vi "Line Datum.vi"(0 "Image in":T2, 1 "Small FOV?":bool, 2 "Angle of rotation":dbl, 3 "half Datum arrow width( in pixels)":u16=50, 4 "Arrow height (in pixels)":u16=50, 5 "Datum origin":cluster{"X":sgl, "Y":sgl}, 6 "Start index":i32=6, 7 "error in (no error)":errorcluster, 8 "Color":u32, 9 "Datum line angle":dbl, 10 "Box start index":i32=1, 12 "sleeping line length(in pixels)":u16=75, 13 "Angular line length(in pixels)":u16=150, 14 "pixel factor":dbl=29160000.0, 15 "Reference string":string="ZAMP", 16 "Measurement name":string, 17 "Fixed overlay details":T1={"Overlay coordinates"=[], "Config coordinates"=[], "Inspection mode?"=TRUE}) -> (20 "Image out":T2, 21 "Text origin out":cluster{"X":sgl, "Y":sgl}, 23 "Overlay coordinates out":cluster{"X":dbl, "Y":dbl}[](array[cluster]), 27 "error out":errorcluster)   [LabVIEW 2019]
uses:
  <vilib>/vision/Image Controls.llb/IMAQ Image.ctl
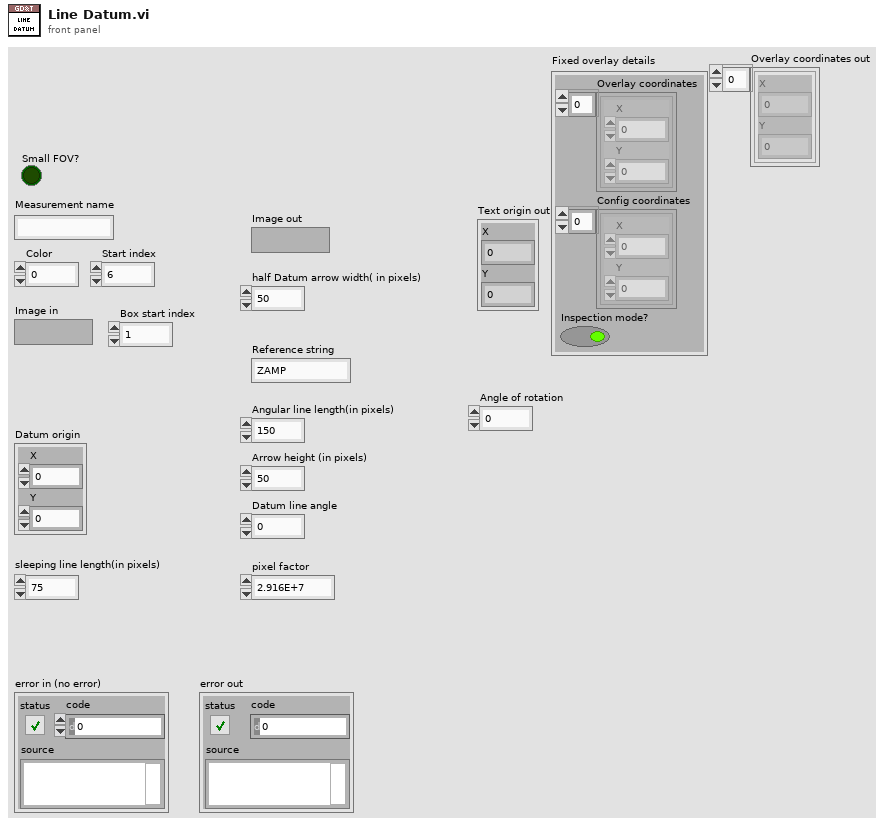
[diagram p1: front panel]
types:
  T1 = cluster{"Overlay coordinates":cluster{"X":dbl, "Y":dbl}[], "Config coordinates":cluster{"X":dbl, "Y":dbl}[], "Inspection mode?":bool}
  T2 = typedef "IMAQ Image.ctl" = refnum<image>
  T3 = enum16{"User-specified Font", "Application Font", "System Font", "Dialog Font"}
  T4 = cluster{"Desired Font (Application)":enum16{"User-specified Font", "Application Font", "System Font", "Dialog Font"}, "[User-specified Font]":cluster{"Font Name":string, "Size":i16, "Strikeout?":bool, "Italic?":bool, "Underline?":bool, "Outline?":bool, "Shadow?":bool, "Bold?":bool, "Rotation Angle":dbl}, "Horizontal Alignment":i16, "Vertical Alignment":i16}
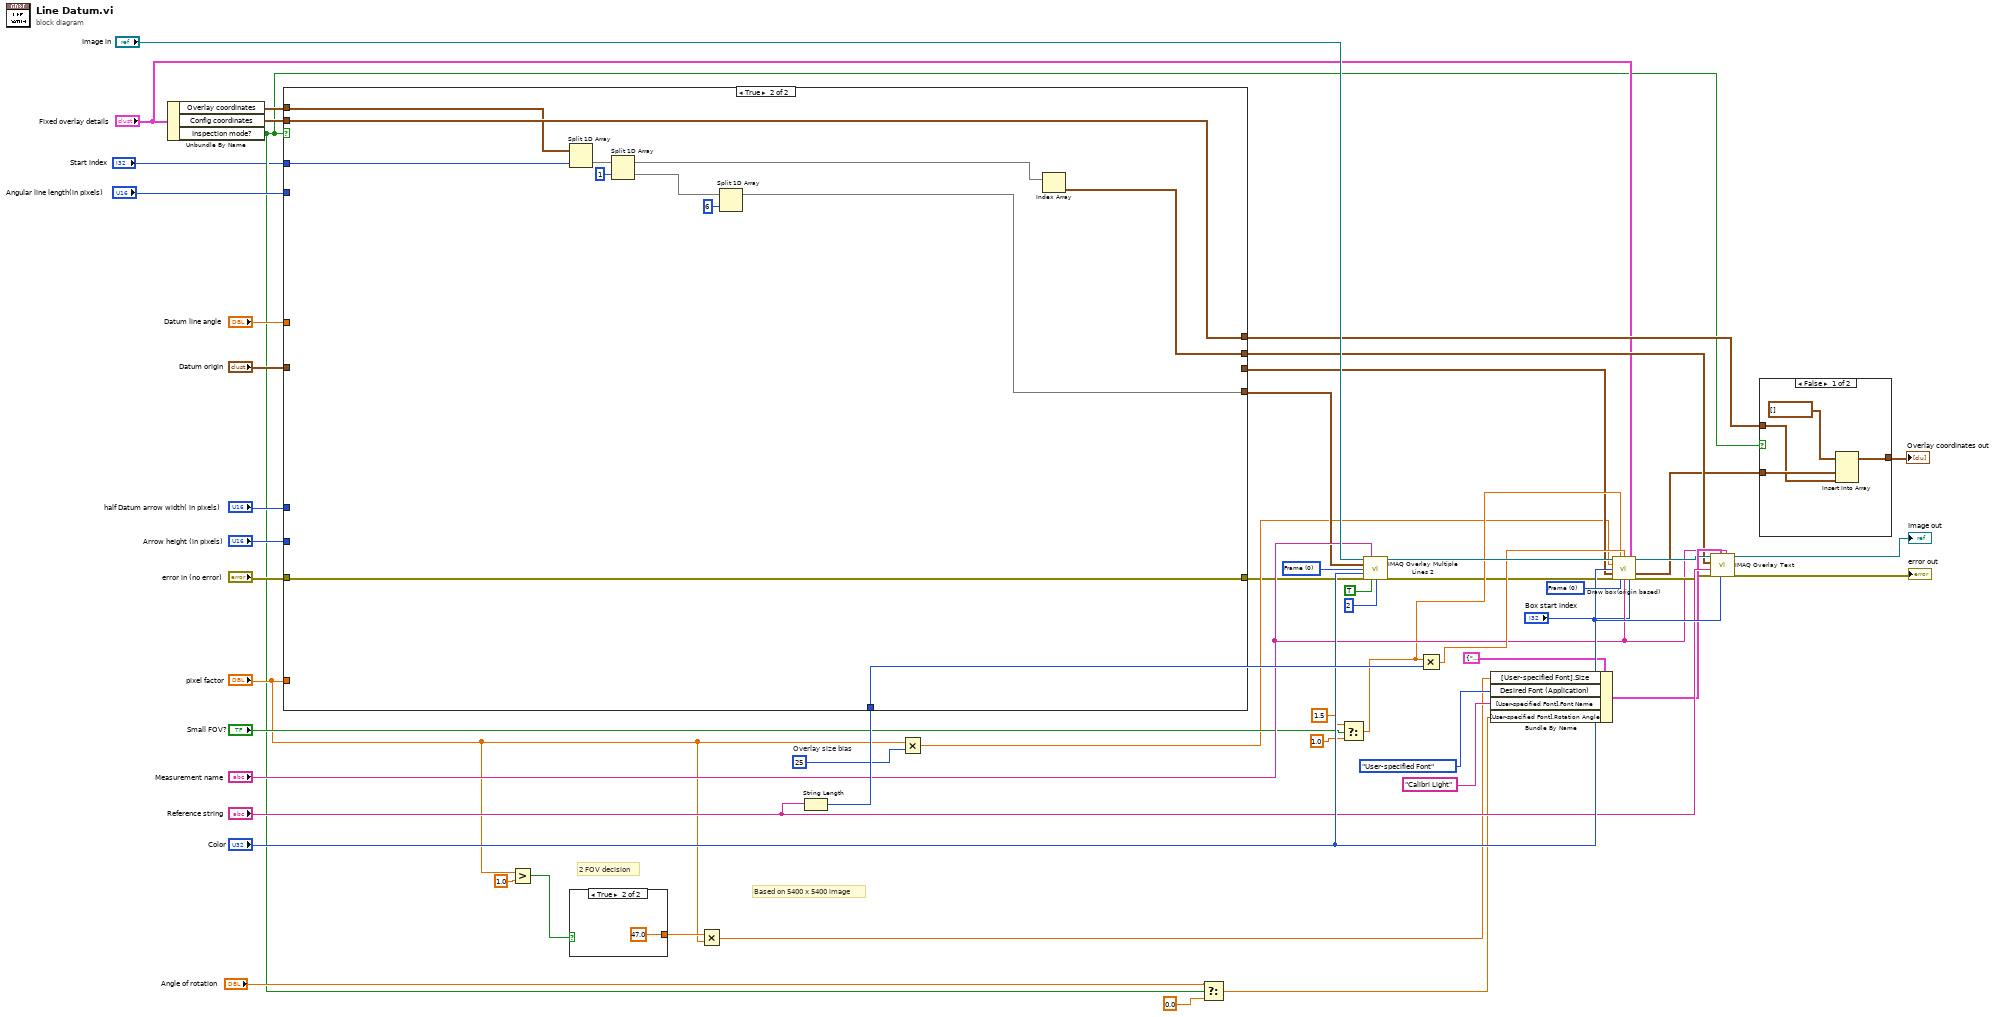
[diagram p0: block diagram]
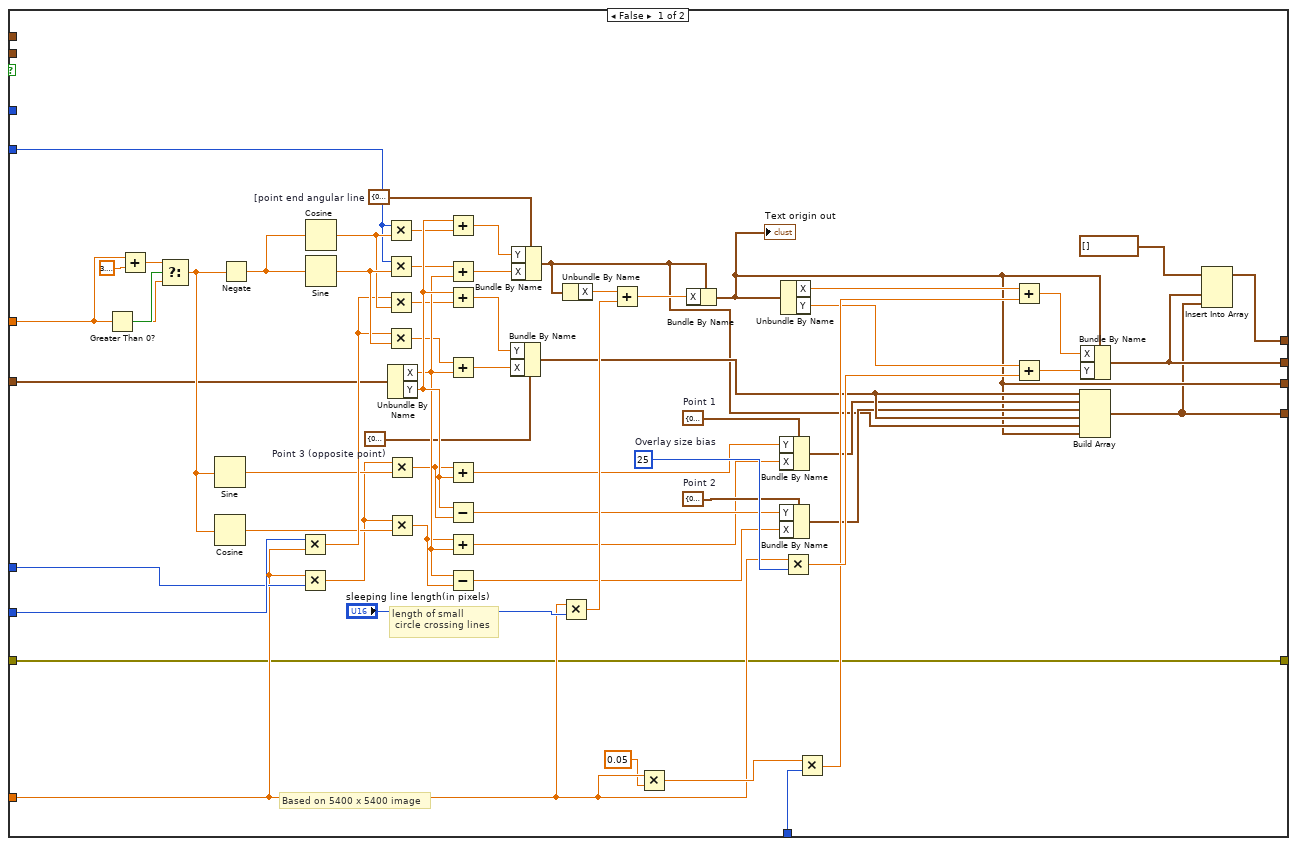
[diagram p3: hidden frame]
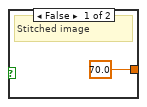
[diagram p4: hidden frame]
diagram:
  w14 = u16 25  # Overlay size bias
  w50 = u32 0 items=["Frame", "Fill"] ("Drawing Mode (Frame)")
  w38 = u32 0 items=["Frame", "Fill"] ("Drawing Mode (Frame)")
  # "2 FOV decision"
  # "Based on 5400 x 5400 image"
  n1 = Unbundle By Name("Fixed overlay details") -> ("Overlay coordinates"=w17:cluster{"X":dbl, "Y":dbl}[], "Config coordinates"=w16:cluster{"X":dbl, "Y":dbl}[], "Inspection mode?"=w4:bool)
  n2 = Greater?(x="pixel factor", y=1.0) -> (0:w35:bool)
  n3 = case shown="True" w35 {
    tunnel: [70.0 ("x") 47.0 ("x")] -> w34
    frame False {
      # "Stitched image"
    }
    frame True {
    }
  }
  n4 = Multiply(x=w34, y="pixel factor") -> (x*y=w28:dbl)
  n5 = String Length(string="Reference string") -> (length=w53:i32)
  n6 = case shown="True" w4 {
    tunnel: w53 -> [w108 _]
    tunnel: "Arrow height (in pixels)" -> [w82 _]
    tunnel: "half Datum arrow width( in pixels)" -> [w80 _]
    tunnel: "Datum origin" -> [w70 _]
    tunnel: "pixel factor" -> [w69 _]
    tunnel: "Angular line length(in pixels)" -> [w68 _]
    tunnel: "Datum line angle" -> [w67 _]
    tunnel: [w56 w119] -> w21
    tunnel: [w59 _] -> w20
    tunnel: [w61 w118] -> w19
    tunnel: w17 -> [_ w126]
    tunnel: w16 -> [_ w127]
    tunnel: [w58 w127] -> w11
    tunnel: "error in (no error)" -> [w57 w123]
    tunnel: [w57 w123] -> w8
    tunnel: "Start index" -> [_ w117]
    frame False {
      w116 = u16 25  # Overlay size bias
      w90 = cluster{"X":sgl, "Y":sgl} {"X"=0.0, "Y"=0.0}  # [point end angular line
      w79 = cluster{"X":sgl, "Y":sgl} {"X"=0.0, "Y"=0.0}  # Point 3 (opposite point)
      w76 = cluster{"X":sgl, "Y":sgl} {"X"=0.0, "Y"=0.0}  # Point 2
      w71 = cluster{"X":sgl, "Y":sgl} {"X"=0.0, "Y"=0.0}  # Point 1
      # "Based on 5400 x 5400 image"
      # "length of small\n circle crossing lines"
      n7 = Greater Than 0?(x=w67) -> (x > 0?=w114:bool)
      n8 = Add(x=w67, y=3.141592653589793) -> (x+y=w112:dbl)
      n9 = Select(t=w112, s=w114, f=w67) -> (s? t:f=w113:dbl)
      n10 = Sine(x=w113) -> (sin(x)=w88:dbl)
      n11 = Cosine(x=w113) -> (cos(x)=w87:dbl)
      n12 = Negate(x=w113) -> (-x=w89:dbl)
      n13 = Multiply(x=w82, y=w69) -> (x*y=w93:dbl)
      n14 = Multiply(x=w69, y=w80) -> (x*y=w81:dbl)
      n15 = Cosine(x=w89) -> (cos(x)=w100:dbl)
      n16 = Sine(x=w89) -> (sin(x)=w101:dbl)
      n17 = Multiply(x=w68, y=w100) -> (x*y=w91:dbl)
      n18 = Multiply(x=w68, y=w101) -> (x*y=w92:dbl)
      n19 = Multiply(x=w93, y=w100) -> (x*y=w86:dbl)
      n20 = Multiply(x=w93, y=w101) -> (x*y=w84:dbl)
      n21 = Multiply(x=w81, y=w88) -> (x*y=w74:dbl)
      n22 = Multiply(x=w81, y=w87) -> (x*y=w75:dbl)
      n23 = Unbundle By Name(w70) -> ("X"=w94:sgl, "Y"=w95:sgl)
      n24 = Add(x=w95, y=w91) -> (x+y=w96:dbl)
      n25 = Add(x=w92, y=w94) -> (x+y=w97:dbl)
      n26 = Add(x=w95, y=w86) -> (x+y=w83:dbl)
      n27 = Add(x=w84, y=w94) -> (x+y=w85:dbl)
      n28 = Add(x=w74, y=w95) -> (x+y=w72:dbl)
      n29 = Subtract(x=w95, y=w74) -> (x-y=w78:dbl)
      n30 = Add(x=w75, y=w94) -> (x+y=w73:dbl)
      n31 = Subtract(x=w94, y=w75) -> (x-y=w77:dbl)
      n32 = Bundle By Name(cluster=w79, "Y"=w83, "X"=w85) -> (w65:cluster{"X":sgl, "Y":sgl})
      n33 = Bundle By Name(cluster=w90, "Y"=w96, "X"=w97) -> (w62:cluster{"X":sgl, "Y":sgl})
      n34 = Multiply(x=w69, y="sleeping line length(in pixels)") -> (x*y=w103:dbl)
      n35 = Unbundle By Name(w62) -> ("X"=w99:sgl)
      n36 = Add(x=w99, y=w103) -> (x+y=w102:dbl)
      n37 = Multiply(x=w69, y=0.05) -> (x*y=w109:dbl)
      n38 = Bundle By Name(cluster=w62, "X"=w102) -> (w59:cluster{"X":sgl, "Y":sgl})
      "Text origin out" <- w59
      n39 = Bundle By Name(cluster=w71, "Y"=w72, "X"=w73) -> (w64:cluster{"X":sgl, "Y":sgl})
      n40 = Bundle By Name(cluster=w76, "Y"=w78, "X"=w77) -> (w63:cluster{"X":sgl, "Y":sgl})
      n41 = Unbundle By Name(w59) -> ("X"=w104:sgl, "Y"=w106:sgl)
      n42 = Multiply(x=w69, y=w116) -> (x*y=w115:dbl)
      n43 = Multiply(x=w109, y=w108) -> (x*y=w110:dbl)
      n44 = Add(x=w104, y=w110) -> (x+y=w105:dbl)
      n45 = Add(x=w106, y=w115) -> (x+y=w107:dbl)
      n46 = Build Array(w65, w64, w63, w65, w62, w59) -> (w56:cluster{"X":sgl, "Y":sgl}[])
      n47 = Bundle By Name(cluster=w59, "X"=w105, "Y"=w107) -> (w61:cluster{"X":sgl, "Y":sgl})
      n48 = Insert Into Array(array=cluster{"X":sgl, "Y":sgl}[] [], new element #1=w61, new element #2=w56) -> (w58:cluster{"X":sgl, "Y":sgl}[])  [unwired: 1 in]
    }
    frame True {
      n49 = Split 1D Array(array=w126, index=w117) -> (second subarray=w125:cluster{"X":dbl, "Y":dbl}[])  [unwired: 1 out]
      n50 = Split 1D Array(array=w125, index=1) -> (first subarray=w124:cluster{"X":dbl, "Y":dbl}[], second subarray=w121:cluster{"X":dbl, "Y":dbl}[])
      n51 = Split 1D Array(array=w121, index=6) -> (first subarray=w119:cluster{"X":dbl, "Y":dbl}[])  [unwired: 1 out]
      n52 = Index Array(array=w124) -> (element=w118:cluster{"X":dbl, "Y":dbl})  [unwired: 1 in]
    }
  }
  n53 = Multiply(x="pixel factor", y=w14) -> (x*y=w13:dbl)
  n54 = Select(t="Angle of rotation", s=w4, f=0.0) -> (s? t:f=w5:dbl)
  n55 = Select(t=1.5, s="Small FOV?", f=1.0 ("Width factor")) -> (s? t:f=w22:dbl)
  n56 = call "IMAQ Overlay Multiple Lines 2"("Image"="Image in", "Group"="Measurement name", "Line End Points"=w21, "Drawing Mode (Frame)"=w38, "Color"="Color", "error in (no error)"=w8, "Maintain Width?"=TRUE, "Width"=u32 2) -> ("Image Out"=w51:T2, "error out"=w18:errorcluster)  [unwired: 6 in]
  n57 = Multiply(x=w22, y=w53) -> (x*y=w44:dbl)
  n58 = Bundle By Name(cluster=T4 {"Desired Font (Application)"=enum."User-specified Font", "[User-specified Font]"={"Font Name"="Calibri Light", "Size"=45, "Strikeout?"=FALSE, "Italic?"=FALSE, "Underline?"=FALSE, "Outline?"=FALSE, "Shadow?"=FALSE, "Bold?"=TRUE, "Rotation Angle"=0.0}, "Horizontal Alignment"=0, "Vertical Alignment"=0} ("Font, Size & Style"), "[User-specified Font].Size"=w28, "Desired Font (Application)"=T3."User-specified Font", "[User-specified Font].Font Name"="Calibri Light", "[User-specified Font].Rotation Angle"=w5) -> (w46:T4)
  n59 = call "Draw box(origin based).vi"("Image"=w51, "Height factor"=w22, "Width factor"=w44, "Fixed overlay details"="Fixed overlay details", "Size bias factor"=w13, "Color Box"="Color", "Origin"=w20, "error in (no error)"=w18, "Drawing Mode (Frame)"=w50, "Group name"="Measurement name", "Start index"="Box start index") -> ("Image Out"=w43:T2, "Overlay coordinates out"=w12:cluster{"X":dbl, "Y":dbl}[], "error out"=w42:errorcluster)  [unwired: 2 out]
  n60 = call "IMAQ Overlay Text"("Group"="Measurement name", "Text Color (black)"="Color", "Font, Size & Style"=w46, "error in (no error)"=w42, "String"="Reference string", "Origin"=w19, "Image"=w43) -> ("error out"=→"error out":errorcluster, "Image Out"=→"Image out":T2)  [unwired: 3 in]
  n61 = case shown="False" w4 {
    tunnel: w12 -> [w131 _]
    tunnel: w11 -> [w130 w132]
    tunnel: [w129 w132] -> w10
    frame False {
      n62 = Insert Into Array(array=cluster{"X":dbl, "Y":dbl}[] [], new element #1=w131, new element #2=w130) -> (w129:cluster{"X":dbl, "Y":dbl}[])  [unwired: 1 in]
    }
    frame True {
    }
  }
  "Overlay coordinates out" <- w10
